vi "katushkakruglaya (3).vi"() -> ()   [LabVIEW 2010]
panel:
  in  "Previous l cursor":bool
  in  "Next l cursor":bool
  in  "Previous R cursor":bool
  in  "Next R cursor":bool
  in  "Значения длины, см":dbl[](array[numeric]) min=0.01 format="%#.2g"
  in  "Значения радиуса, см":dbl[](array[numeric]) min=0.01 format="%#.2g"
  in  "stop":bool
  out "L(n) при R = const":dbl[][](graph)
  out "L(n) при l = const":dbl[][](graph)
  in  "Индуктивность L, нГн":dbl=1359.627 min=0.0 format="%#.3g"
  in  "Длина катушки l, см":dbl=2.0 min=0.0 format="%#.3g"
  out "Число витков, n":dbl
  in  "Радиус катушки R, см":dbl=1.0 min=0.001 format="%#.3g"
  # "Программа расчёта числа витков однослойной катушки круглого сечения"
  # "Формула для расчёта индуктивности \nоднослойной катушки круглого сечения:"
  # "Остановить работу\nпрограммы:"
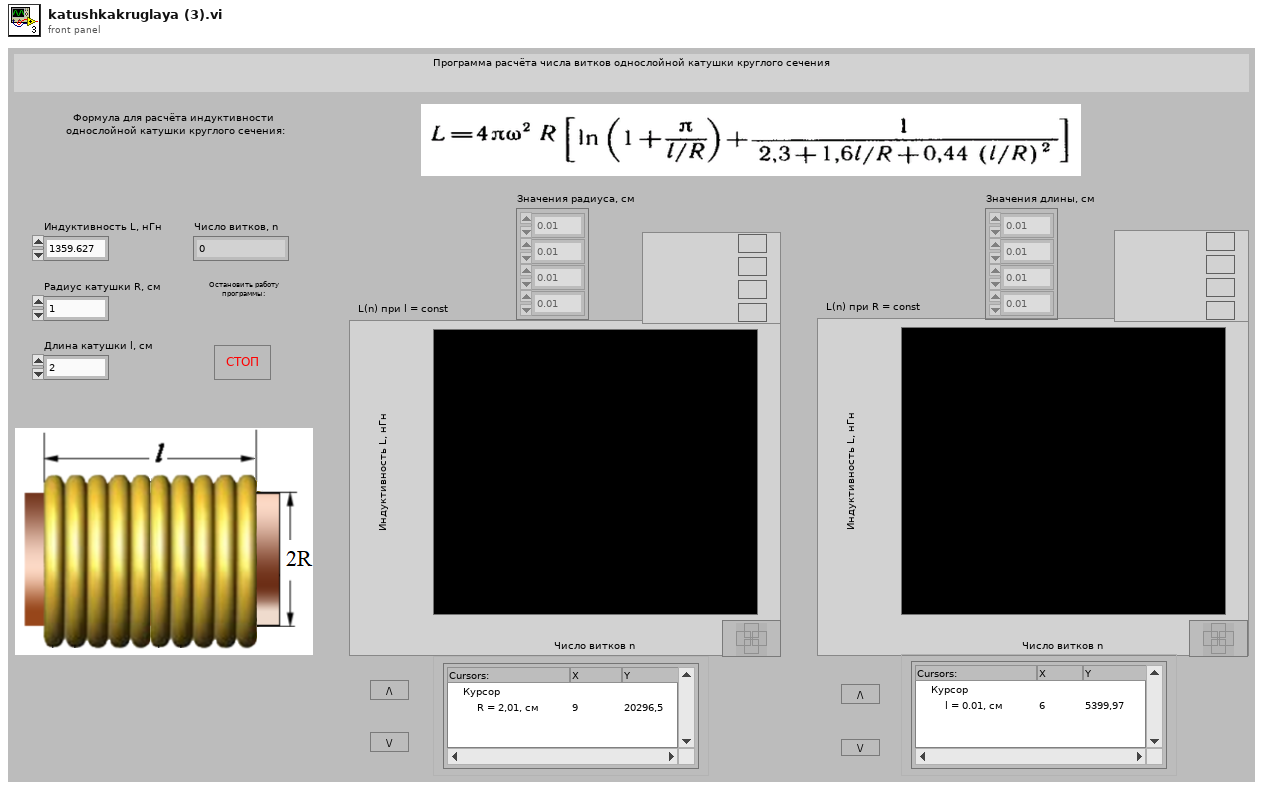
[diagram p1: front panel]
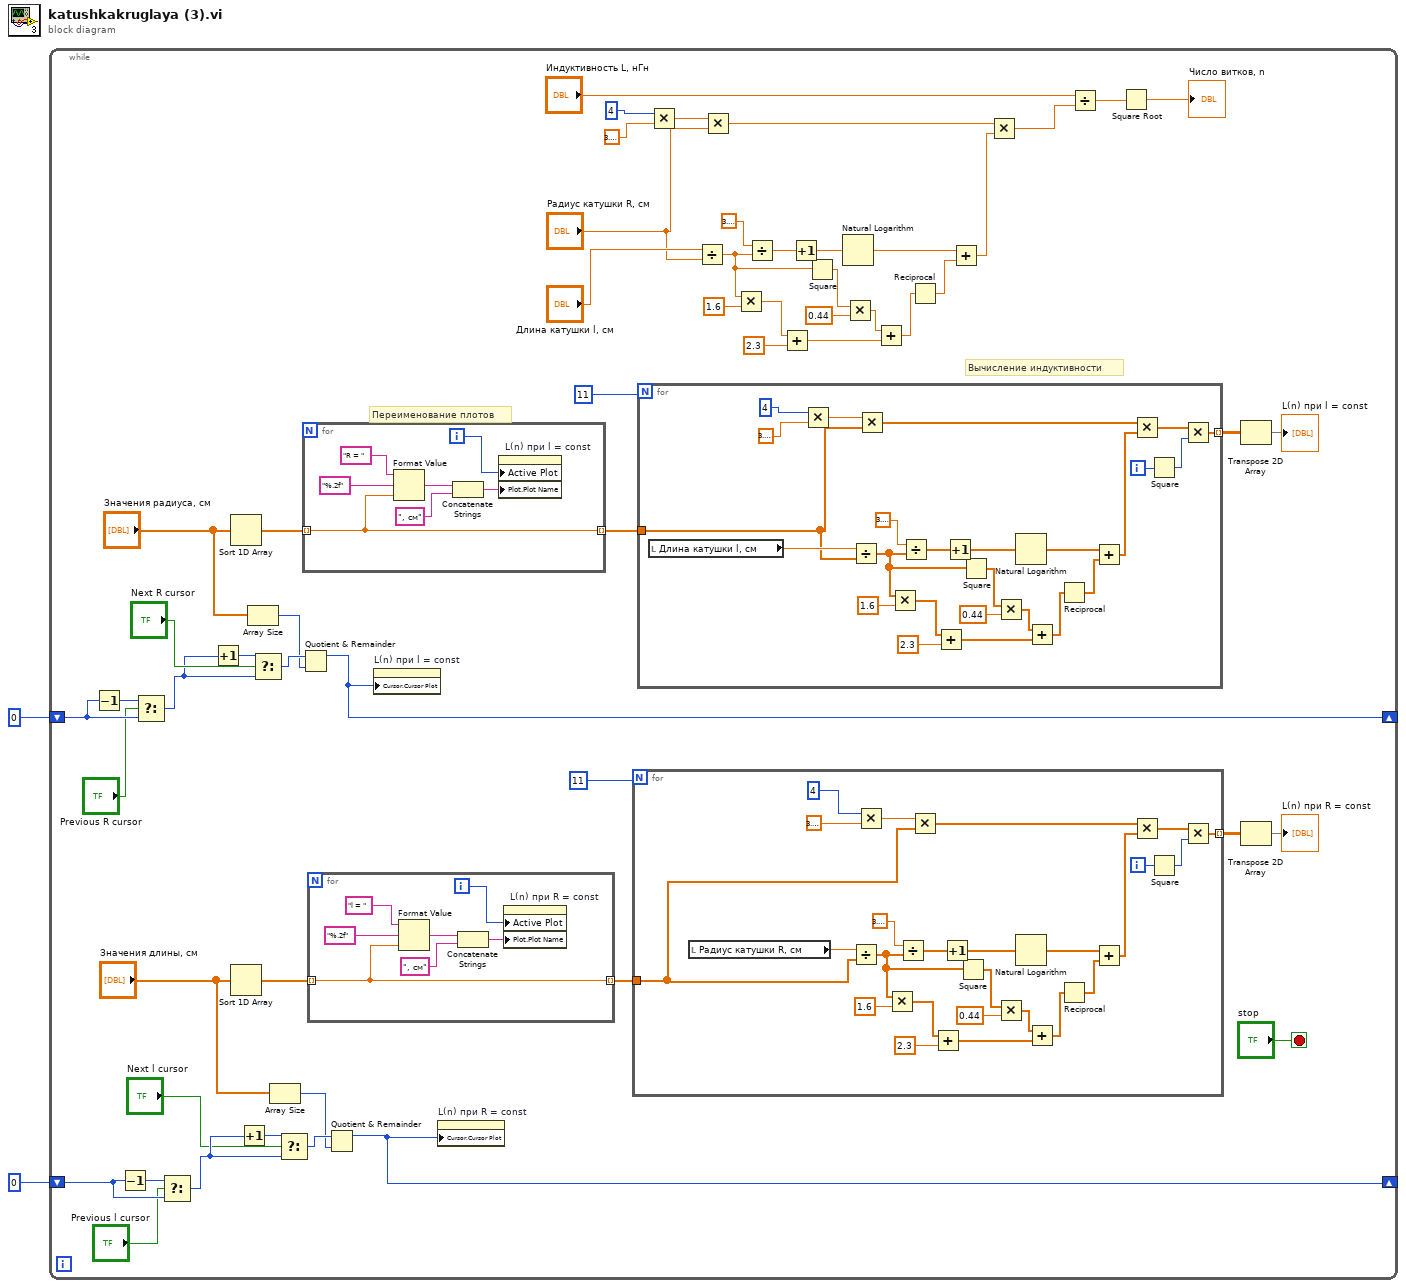
[diagram p0: block diagram]
diagram:
  n1 = while {
    shift-right: [w17] -> _
    shift-left: 0 ("Cursor.Cursor Plot") -> [w14]
    shift-right: [w5] -> _
    shift-left: 0 ("Cursor.Cursor Plot") -> [w8]
    stop <- "stop" stop-if-true
    # "Вычисление индуктивности"
    # "Переименование плотов"
    n2 = Decrement(x=w14) -> (x-1=w15:i32)
    n3 = Decrement(x=w8) -> (x-1=w9:i32)
    n4 = Select(t=w15, s="Previous R cursor", f=w14) -> (s? t:f=w16:i32)
    n5 = Select(t=w9, s="Previous l cursor", f=w8) -> (s? t:f=w10:i32)
    n6 = Increment(x=w16) -> (x+1=w21:i32)
    n7 = Sort 1D Array(array="Значения радиуса, см") -> (sorted array=w25:dbl[])
    n8 = Sort 1D Array(array="Значения длины, см") -> (sorted array=w24:dbl[])
    n9 = Increment(x=w10) -> (x+1=w12:i32)
    n10 = Array Size(array="Значения радиуса, см") -> (size(s)=w18:i32)
    n11 = Select(t=w21, s="Next R cursor", f=w16) -> (s? t:f=w19:i32)
    n12 = Array Size(array="Значения длины, см") -> (size(s)=w3:i32)
    n13 = Select(t=w12, s="Next l cursor", f=w10) -> (s? t:f=w11:i32)
    n14 = Quotient & Remainder(x=w19, y=w18) -> (x-y*floor(x/y)=w17:i32)  [unwired: 1 out]
    n15 = for {
      tunnel: w25 -> [w71] mode=indexing
      tunnel: [w71] -> w27 mode=indexing
      i -> [w72]
      n16 = Format Value(string ("")="R = ", format string="%.2f", value (0)=w71) -> (output string=w69:string)
      n17 = Concatenate Strings(w69, ", см") -> (w68:string)
      n18 = property on="L(n) при l = const" class="WFGraph (strict)"("Active Plot"=w72, "Plot.Plot Name"=w68) -> ()  [unwired: 2 in, 2 out]
    }
    n19 = for {
      tunnel: w24 -> [w64] mode=indexing
      tunnel: [w64] -> w23 mode=indexing
      i -> [w65]
      n20 = Format Value(string ("")="l = ", format string="%.2f", value (0)=w64) -> (output string=w62:string)
      n21 = Concatenate Strings(w62, ", см") -> (w61:string)
      n22 = property on="L(n) при R = const" class="WFGraph (strict)"("Active Plot"=w65, "Plot.Plot Name"=w61) -> ()  [unwired: 2 in, 2 out]
    }
    n23 = Quotient & Remainder(x=w11, y=w3) -> (x-y*floor(x/y)=w5:i32)  [unwired: 1 out]
    n24 = property on="L(n) при l = const" class="WFGraph (strict)"("Cursor.Cursor Plot"=w17) -> ()  [unwired: 2 in, 2 out]
    n25 = property on="L(n) при R = const" class="WFGraph (strict)"("Cursor.Cursor Plot"=w5) -> ()  [unwired: 2 in, 2 out]
    n26 = for {
      N: 11 -> [_]
      tunnel: [w76] -> w29 mode=indexing
      tunnel: w23 -> [w74]
      i -> [w73]
      n27 = local read "Радиус катушки R, см"() -> (w75:dbl)
      n28 = Divide(x=w75, y=w74) -> (x/y=w84:dbl[])
      n29 = Multiply(x=4, y=3.141592653589793) -> (x*y=w95:dbl)
      n30 = Multiply(x=w84, y=1.6) -> (x*y=w88:dbl[])
      n31 = Divide(x=3.141592653589793, y=w84) -> (x/y=w90:dbl[])
      n32 = Multiply(x=w95, y=w74) -> (x*y=w82:dbl[])
      n33 = Add(x=w88, y=2.3) -> (x+y=w86:dbl[])
      n34 = Increment(x=w90) -> (x+1=w94:dbl[])
      n35 = Square(x=w84) -> (x^2=w81:dbl[])
      n36 = Multiply(x=w81, y=0.44) -> (x*y=w80:dbl[])
      n37 = Natural Logarithm(1:w94) -> (0:w93:dbl[])
      n38 = Add(x=w80, y=w86) -> (x+y=w85:dbl[])
      n39 = Reciprocal(x=w85) -> (1/x=w92:dbl[])
      n40 = Add(x=w93, y=w92) -> (x+y=w83:dbl[])
      n41 = Multiply(x=w82, y=w83) -> (x*y=w78:dbl[])
      n42 = Square(x=w73) -> (x^2=w77:i32)
      n43 = Multiply(x=w78, y=w77) -> (x*y=w76:dbl[])
    }
    n44 = for {
      N: 11 -> [_]
      tunnel: [w103] -> w32 mode=indexing
      tunnel: w27 -> [w101]
      i -> [w98]
      n45 = local read "Длина катушки l, см"() -> (w102:dbl)
      n46 = Multiply(x=4, y=3.141592653589793) -> (x*y=w120:dbl)
      n47 = Divide(x=w102, y=w101) -> (x/y=w109:dbl[])
      n48 = Multiply(x=w120, y=w101) -> (x*y=w107:dbl[])
      n49 = Multiply(x=w109, y=1.6) -> (x*y=w113:dbl[])
      n50 = Divide(x=3.141592653589793, y=w109) -> (x/y=w115:dbl[])
      n51 = Add(x=w113, y=2.3) -> (x+y=w111:dbl[])
      n52 = Increment(x=w115) -> (x+1=w119:dbl[])
      n53 = Square(x=w109) -> (x^2=w106:dbl[])
      n54 = Multiply(x=w106, y=0.44) -> (x*y=w105:dbl[])
      n55 = Natural Logarithm(1:w119) -> (0:w118:dbl[])
      n56 = Add(x=w105, y=w111) -> (x+y=w110:dbl[])
      n57 = Reciprocal(x=w110) -> (1/x=w117:dbl[])
      n58 = Add(x=w118, y=w117) -> (x+y=w108:dbl[])
      n59 = Multiply(x=w107, y=w108) -> (x*y=w99:dbl[])
      n60 = Square(x=w98) -> (x^2=w100:i32)
      n61 = Multiply(x=w99, y=w100) -> (x*y=w103:dbl[])
    }
    n62 = Multiply(x=4, y=3.141592653589793) -> (x*y=w56:dbl)
    n63 = Divide(x="Длина катушки l, см", y="Радиус катушки R, см") -> (x/y=w43:dbl)
    n64 = Multiply(x=w56, y="Радиус катушки R, см") -> (x*y=w40:dbl)
    n65 = Multiply(x=w43, y=1.6) -> (x*y=w47:dbl)
    n66 = Divide(x=3.141592653589793, y=w43) -> (x/y=w49:dbl)
    n67 = Add(x=w47, y=2.3) -> (x+y=w45:dbl)
    n68 = Increment(x=w49) -> (x+1=w55:dbl)
    n69 = Square(x=w43) -> (x^2=w38:dbl)
    n70 = Natural Logarithm(1:w55) -> (0:w54:dbl)
    n71 = Multiply(x=w38, y=0.44) -> (x*y=w37:dbl)
    n72 = Add(x=w37, y=w45) -> (x+y=w44:dbl)
    n73 = Reciprocal(x=w44) -> (1/x=w53:dbl)
    n74 = Add(x=w54, y=w53) -> (x+y=w41:dbl)
    n75 = Multiply(x=w40, y=w41) -> (x*y=w42:dbl)
    n76 = Divide(x="Индуктивность L, нГн", y=w42) -> (x/y=w39:dbl)
    n77 = Square Root(x=w39) -> (sqrt(x)=→"Число витков, n":dbl)
    n78 = Transpose 2D Array(2D array=w32) -> (transposed array=→"L(n) при l = const":dbl[][])
    n79 = Transpose 2D Array(2D array=w29) -> (transposed array=→"L(n) при R = const":dbl[][])
  }
